vi "TreeNode Put Row.vi"(0 "TreeNode DVR in":refnum<data-value>, 5 "Row Data":refnum<data-value>, 7 "Time":i64, 9 "Size (1024)":i32=1024, 11 "error in (no error)":errorcluster) -> (4 "TreeNode DVR out":refnum<data-value>, 15 "error out":errorcluster)   [LabVIEW 2015, in "MDSplus.lvlib"]
doc: "Write a single row of timestamped data."
uses:
  MDSplus.lvlib
  Classes/Data_Class/TreeNode_Class/TreeNode.lvclass
  Classes/Data_Class/Data.lvclass
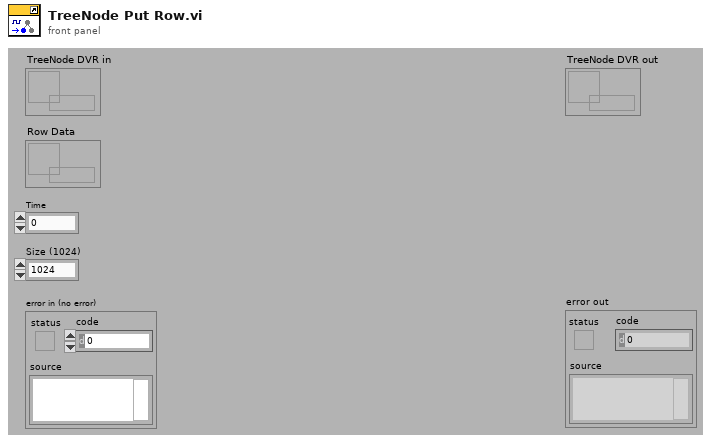
[diagram p1: front panel]
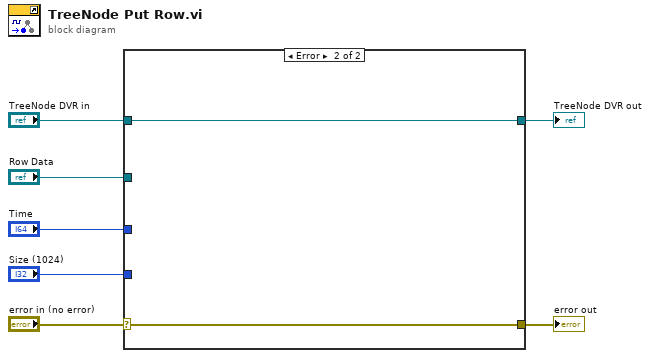
[diagram p0: block diagram]
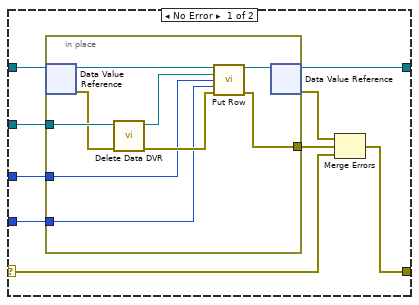
[diagram p2: hidden frame]
diagram:
  n1 = case shown="Error" "error in (no error)" {
    selector: "error in (no error)" -> [w15 w26]
    tunnel: "TreeNode DVR in" -> [w16 w27]
    tunnel: [w12 w26] -> w7
    tunnel: [w13 w27] -> w4
    tunnel: "Row Data" -> [w10 _]
    tunnel: "Time" -> [w9 _]
    tunnel: "Size (1024)" -> [w8 _]
    frame No Error {
      n2 = in-place {
        in-place-border: [w19] -> w11
        in-place-border: w10 -> [w23]
        in-place-border: w9 -> [w18]
        in-place-border: w8 -> [w17]
        n3 = in-place-dvr #1(w16) -> (w25:refnum<class "TreeNode.lvclass">, w22:errorcluster)
        n4 = call "Delete Data DVR.vi"("error in (no error)"=w22, "Data DVR in"=w23) -> ("error out"=w21:errorcluster, "Data out"=w20:refnum<class "Data.lvclass">)  [unwired: 8 in]
        n5 = call-dynamic "Put Row.vi"("TreeNode in"=w25, "Row data"=w20, "Time"=w18, "Size (1024)"=w17, "error in (no error)"=w21) -> ("TreeNode out"=w24:refnum<class "TreeNode.lvclass">, "error out"=w19:errorcluster)  [unwired: 9 in]
        n6 = in-place-dvr #1(w24) -> (w13:refnum<data-value>, w14:errorcluster)
      }
      n7 = Merge Errors(w14, w11, w15) -> (w12:errorcluster)
    }
    frame Error {
    }
  }
  "error out" <- w7
  "TreeNode DVR out" <- w4
